vi "demo.vi"() -> ()   [LabVIEW 2015]
panel:
  out "Meter":dbl(knob) scale=0.0..10.0
  in  "Numeric 2":dbl
  in  "Numeric":dbl
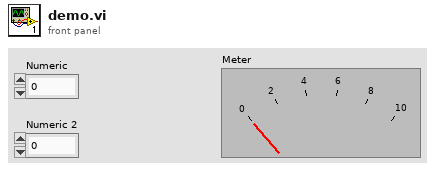
[diagram p1: front panel]
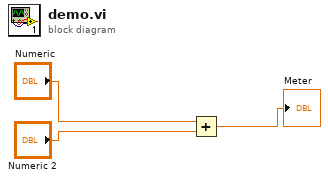
[diagram p0: block diagram]
diagram:
  n1 = Add(x="Numeric", y="Numeric 2") -> (x+y=→"Meter":dbl)
